vi "Read Iteration Count.vi"(8 "error in (no error)":errorcluster, 11 "Function in":refnum<class "Function.lvclass">) -> (0 "error out":errorcluster, 2 "Iteration Count":T1, 3 "Function out":refnum<class "Function.lvclass">)   [LabVIEW 2016]
uses:
  <userlib>/Common Components/Function Actor/Function.lvclass
  C:/Program Files (x86)/National Instruments/LabVIEW 2016/vi.lib/ActorFramework/Actor/Actor.lvclass
  <userlib>/Common Components/Function Actor/Iteration Count.ctl
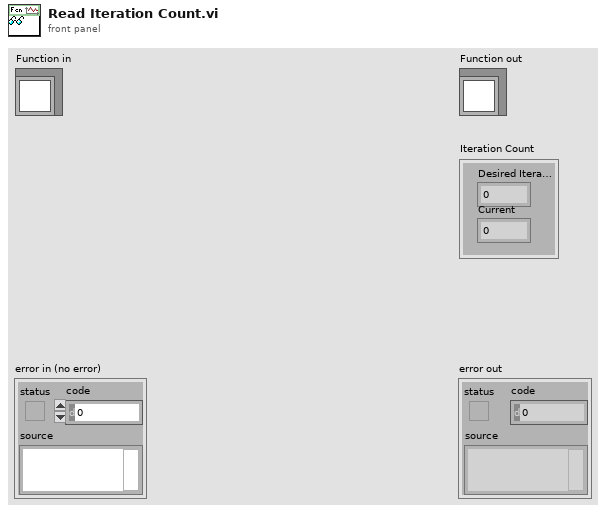
[diagram p1: front panel]
types:
  T1 = typedef "Iteration Count.ctl" = cluster{"Desired Iterations":i32, "Current":i32}
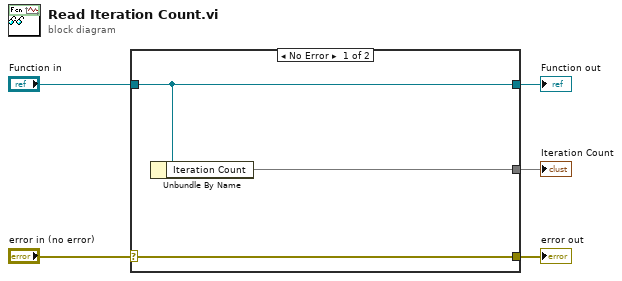
[diagram p0: block diagram]
diagram:
  n1 = case shown="No Error" "error in (no error)" {
    selector: "error in (no error)" -> [w8 w9]
    tunnel: [w8 w9] -> w4
    tunnel: [w7 w10] -> w2
    tunnel: "Function in" -> [w7 w10]
    tunnel: [w6 _] -> w1
    frame No Error {
      n2 = Unbundle By Name(w7) -> ("Iteration Count"=w6)
    }
    frame Error {
    }
  }
  "error out" <- w4
  "Function out" <- w2
  "Iteration Count" <- w1
